vi "Configure TDMS.vi"(8 "error in (no error)":errorcluster, 11 "DataLogger in":refnum<class "DataLogger.lvclass">) -> (0 "error out":errorcluster, 3 "DataLogger out":refnum<class "DataLogger.lvclass">)   [LabVIEW 2020, in "VolatusDataLogger.lvlib" / "DataLogger.lvclass"]
uses:
  DataLogger.lvclass
  DataLogger.lvclass/DataLogger.ctl
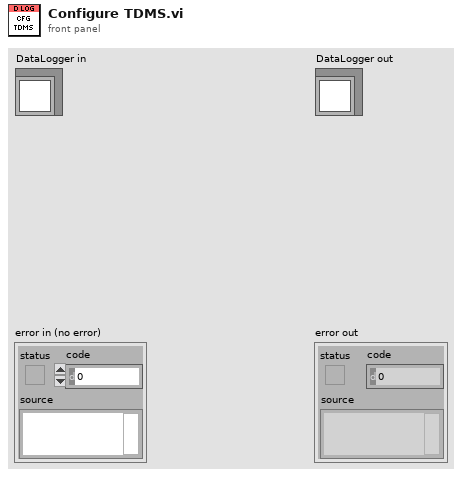
[diagram p1: front panel]
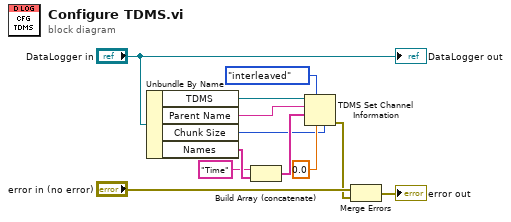
[diagram p0: block diagram]
diagram:
  n1 = Unbundle By Name("DataLogger in") -> ("TDMS"=w5:refnum<k34>, "Parent Name"=w7:string, "Chunk Size"=w3:u32, "Names"=w10:string[])
  n2 = Build Array (concatenate)("Time", w10) -> (w8:string[])
  n3 = TDMS Set Channel Information(4:w3, 6:0.0, 7:enum16{"non-interleaved", "interleaved"}."interleaved" ("data layout (0:non-interleaved)"), 9:w8, 10:w7, 11:w5) -> (0:w1:errorcluster)  [unwired: 1 in, 1 out]
  n4 = Merge Errors("error in (no error)", w1) -> (→"error out":errorcluster)
  "DataLogger out" <- "DataLogger in"
